vi "Scale Adjustment Menu.vi"(8 "error in":errorcluster, 11 "Data Frame Format":T1) -> (0 "Scale Minimum":dbl, 1 "Scale Maximum":dbl, 2 "Active Y scale":u32, 3 "Request Cancelled":bool, 4 "error out":errorcluster)   [LabVIEW 2015]
doc: "Adjustment menu for manually setting the chart scales for a desired variable. Used in the \"Alicat Full Example\" VI"
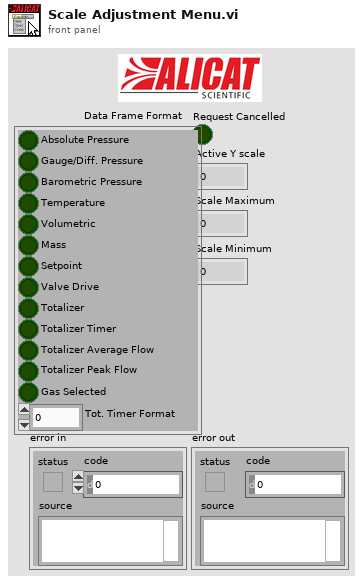
[diagram p1: front panel]
types:
  T1 = cluster{"Absolute Pressure":bool, "Gauge/Diff. Pressure":bool, "Barometric Pressure":bool, "Temperature":bool, "Volumetric":bool, "Mass":bool, "Setpoint":bool, "Valve Drive":bool, "Totalizer":bool, "Totalizer Timer":bool, "Totalizer Average Flow":bool, "Totalizer Peak Flow":bool, "Gas Selected":bool, "Tot. Timer Format":u16}
  T2 = enum16{"Left Button", "Center Button", "Right Button", "Window Close"}
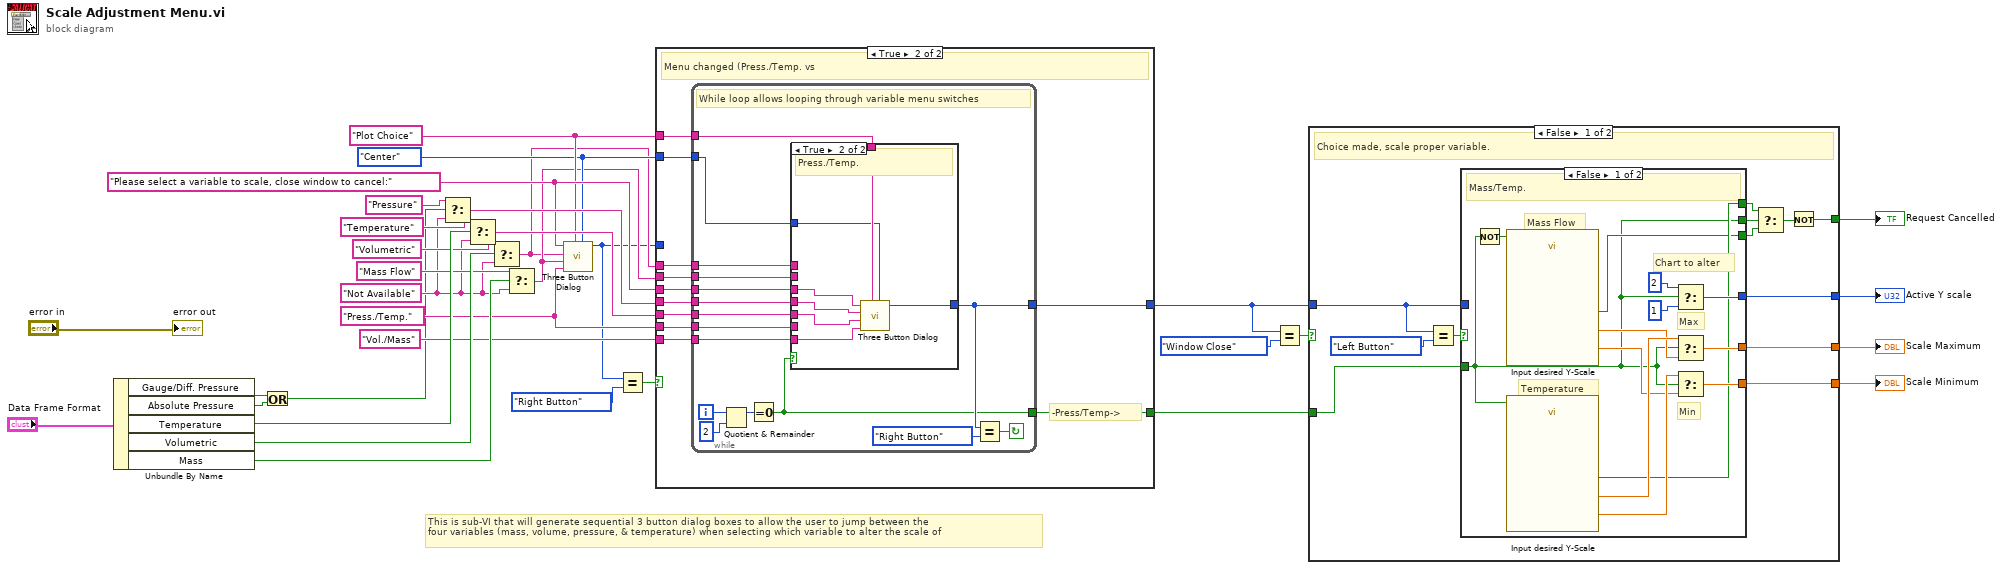
[diagram p0: block diagram]
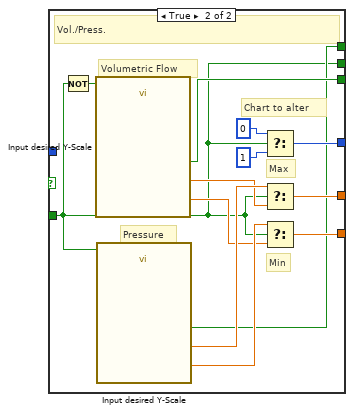
[diagram p2: hidden frame]
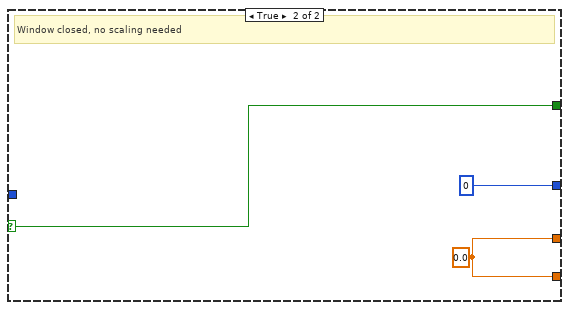
[diagram p3: hidden frame]
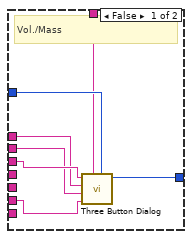
[diagram p5: hidden frame]
diagram:
  w20 = enum16{"Left", "Center", "Right"}."Center" ("Justify Message (Left)")
  w17 = "Press./Temp." ("Right Button Text (\"Cancel\")")
  w26 = "Not Available" ("Right Button Text (\"Cancel\")")
  w21 = "Plot Choice" ("message")
  w22 = "Please select a variable to scale, close window to cancel:" ("message")
  # "This is sub-VI that will generate sequential 3 button dialog boxes to allow the user to jump between the\nfour variables (mass, volume, pressure, & temperature) when selecting which variable to alter the scale of"
  n1 = Unbundle By Name("Data Frame Format") -> ("Gauge/Diff. Pressure"=w4:bool, "Absolute Pressure"=w3:bool, "Temperature"=w31:bool, "Volumetric"=w29:bool, "Mass"=w27:bool)
  n2 = Or(x=w4, y=w3) -> (x .or. y?=w2:bool)
  n3 = Select(t="Pressure" ("Right Button Text (\"Cancel\")"), s=w2, f=w26) -> (s? t:f=w25:string)
  n4 = Select(t="Temperature" ("Right Button Text (\"Cancel\")"), s=w31, f=w26) -> (s? t:f=w24:string)
  n5 = Select(t="Volumetric" ("Right Button Text (\"Cancel\")"), s=w29, f=w26) -> (s? t:f=w15:string)
  n6 = Select(t="Mass Flow" ("Right Button Text (\"Cancel\")"), s=w27, f=w26) -> (s? t:f=w16:string)
  n7 = call <vilib>:"Three Button Dialog.vi"("Justify Message (Left)"=w20, "Window Title (\"\")"=w21, "Right Button Text (\"Cancel\")"=w17, "Center Button Text (\"No\")"=w16, "Left Button Text (\"Yes\")"=w15, "message"=w22) -> ("Which Button?"=w10:T2)  [unwired: 5 in]
  n8 = Equal?(x=w10, y=T2."Right Button" ("Which Button?")) -> (x = y?=w19:bool)
  n9 = case shown="True" w19 {
    selector: w19 -> [w35 _]
    tunnel: w25 -> [_ w46]
    tunnel: w24 -> [_ w45]
    tunnel: "Vol./Mass" ("Right Button Text (\"Cancel\")") -> [_ w44]
    tunnel: w22 -> [_ w43]
    tunnel: w21 -> [_ w42]
    tunnel: w20 -> [_ w41]
    tunnel: [w34 w37] -> w11
    tunnel: w17 -> [_ w38]
    tunnel: w16 -> [_ w40]
    tunnel: w15 -> [_ w39]
    tunnel: [w35 w36] -> w14
    tunnel: w10 -> [w34 _]
    frame False {
      # "Selection made or window closed"
    }
    frame True {
      # "-Press/Temp->"
      # "Menu changed (Press./Temp. vs"
      n10 = while {
        tunnel: w46 -> [w62]
        tunnel: w45 -> [w61]
        tunnel: w44 -> [w60]
        tunnel: w43 -> [w59]
        tunnel: w42 -> [w58]
        tunnel: w41 -> [w57]
        tunnel: w40 -> [w51]
        tunnel: w39 -> [w50]
        tunnel: w38 -> [w49]
        tunnel: [w48] -> w37
        tunnel: [w47] -> w36
        i -> [w56]
        stop <- w52 continue-if-true
        # "While loop allows looping through variable menu switches"
        n11 = Quotient & Remainder(x=w56, y=2) -> (x-y*floor(x/y)=w54:i32)  [unwired: 1 out]
        n12 = Equal To 0?(x=w54) -> (x = 0?=w47:bool)
        n13 = case shown="True" w47 {
          tunnel: w62 -> [_ w76]
          tunnel: w61 -> [_ w75]
          tunnel: w60 -> [_ w74]
          tunnel: w59 -> [w68 w73]
          tunnel: w58 -> [w63 w72]
          tunnel: w57 -> [w64 w71]
          tunnel: [w69 w70] -> w48
          tunnel: w51 -> [w65 _]
          tunnel: w50 -> [w66 _]
          tunnel: w49 -> [w67 _]
          frame False {
            # "Vol./Mass"
            n14 = call <vilib>:"Three Button Dialog.vi"("Justify Message (Left)"=w64, "Window Title (\"\")"=w63, "Right Button Text (\"Cancel\")"=w67, "Center Button Text (\"No\")"=w65, "Left Button Text (\"Yes\")"=w66, "message"=w68) -> ("Which Button?"=w69:T2)  [unwired: 5 in]
          }
          frame True {
            # "Press./Temp."
            n15 = call <vilib>:"Three Button Dialog.vi"("Justify Message (Left)"=w71, "Window Title (\"\")"=w72, "Right Button Text (\"Cancel\")"=w74, "Center Button Text (\"No\")"=w75, "Left Button Text (\"Yes\")"=w76, "message"=w73) -> ("Which Button?"=w70:T2)  [unwired: 5 in]
          }
        }
        n16 = Equal?(x=w48, y=T2."Right Button" ("Which Button?")) -> (x = y?=w52:bool)
      }
    }
  }
  n17 = Equal?(x=w11, y=T2."Window Close" ("Which Button?")) -> (x = y?=w12:bool)
  n18 = case shown="False" w12 {
    selector: w12 -> [_ w116]
    tunnel: w11 -> [w87 _]
    tunnel: w14 -> [w85 _]
    tunnel: [w84 w117] -> w6
    tunnel: [w83 w117] -> w7
    tunnel: [w77 w116] -> w9
    tunnel: [w82 u32 0] -> w8
    frame False {
      # "Choice made, scale proper variable."
      n19 = Equal?(x=w87, y=T2."Left Button" ("Which Button?")) -> (x = y?=w86:bool)
      n20 = case shown="False" w86 {
        tunnel: w87 -> [_ _]
        tunnel: w85 -> [w89 w102]
        tunnel: [w97 w108] -> w83
        tunnel: [w96 w109] -> w84
        tunnel: [w98 w105] -> w82
        tunnel: [w90 w104] -> w80
        tunnel: [w91 w103] -> w79
        tunnel: [w89 w102] -> w81
        frame False {
          # "Min"
          # "Max"
          # "Chart to alter"
          # "Mass Flow"
          # "Temperature"
          # "Mass/Temp."
          n21 = Not(x=w89) -> (.not. x?=w101:bool)
          n22 = call "Input desired Y-Scale"("Enable"=w101) -> ("Scale Minimum"=w92:dbl, "Scale Maximum"=w93:dbl, "OK"=w90:bool)  [unwired: 15 in, 1 out]
          n23 = call "Input desired Y-Scale"("Enable"=w89) -> ("Scale Minimum"=w95:dbl, "Scale Maximum"=w94:dbl, "OK"=w91:bool)  [unwired: 15 in, 1 out]
          n24 = Select(t=u32 2, s=w89, f=u32 1) -> (s? t:f=w98:u32)
          n25 = Select(t=w94, s=w89, f=w93) -> (s? t:f=w97:dbl)
          n26 = Select(t=w95, s=w89, f=w92) -> (s? t:f=w96:dbl)
        }
        frame True {
          # "Min"
          # "Max"
          # "Chart to alter"
          # "Pressure"
          # "Volumetric Flow"
          # "Vol./Press."
          n27 = Not(x=w102) -> (.not. x?=w114:bool)
          n28 = call "Input desired Y-Scale"("Enable"=w114) -> ("Scale Minimum"=w110:dbl, "Scale Maximum"=w111:dbl, "OK"=w104:bool)  [unwired: 15 in, 1 out]
          n29 = call "Input desired Y-Scale"("Enable"=w102) -> ("Scale Minimum"=w112:dbl, "Scale Maximum"=w113:dbl, "OK"=w103:bool)  [unwired: 15 in, 1 out]
          n30 = Select(t=u32 0, s=w102, f=u32 1) -> (s? t:f=w105:u32)
          n31 = Select(t=w113, s=w102, f=w111) -> (s? t:f=w108:dbl)
          n32 = Select(t=w112, s=w102, f=w110) -> (s? t:f=w109:dbl)
        }
      }
      n33 = Select(t=w79, s=w81, f=w80) -> (s? t:f=w78:bool)
      n34 = Not(x=w78) -> (.not. x?=w77:bool)
    }
    frame True {
      w117 = 0.0 ("Scale Maximum")
      # "Window closed, no scaling needed"
    }
  }
  "Request Cancelled" <- w9
  "Active Y scale" <- w8
  "Scale Maximum" <- w7
  "Scale Minimum" <- w6
  "error out" <- "error in"
